vi "延时2.vi"() -> ()   [LabVIEW 2017]
panel:
  out "t2":u32
  in  "t1":u32
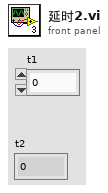
[diagram p1: front panel]
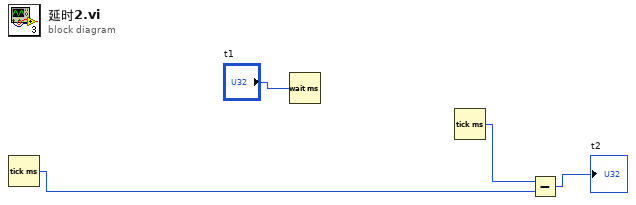
[diagram p0: block diagram]
diagram:
  n1 = Tick Count (ms)() -> (millisecond timer value=w3:u32)
  n2 = Wait (ms)(milliseconds to wait="t1") -> ()  [unwired: 1 out]
  n3 = Tick Count (ms)() -> (millisecond timer value=w4:u32)
  n4 = Subtract(x=w4, y=w3) -> (x-y=→"t2":u32)
